vi "MTS_AutoZPos.vi"(0 "PH Dev":i32, 1 "OFlow Interv [s]":dbl, 2 "Accum Time [s]":dbl=0.1, 5 "PI System no.":i32, 11 "error in":errorcluster, 12 "Start Point":T1, 13 "Steps":i32=9, 14 "Step Width [um]":dbl=0.5) -> (4 "New Z":dbl, 6 "Counts":u32[](array[numeric]), 15 "error out":errorcluster)   [LabVIEW 2010]
panel:
  out "FiFo Overrun":bool
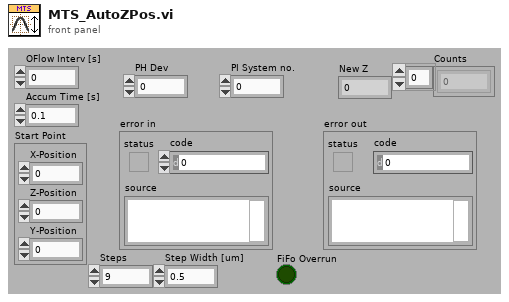
[diagram p1: front panel]
types:
  T1 = cluster{"X-Position":dbl, "Y-Position":dbl, "Z-Position":dbl}
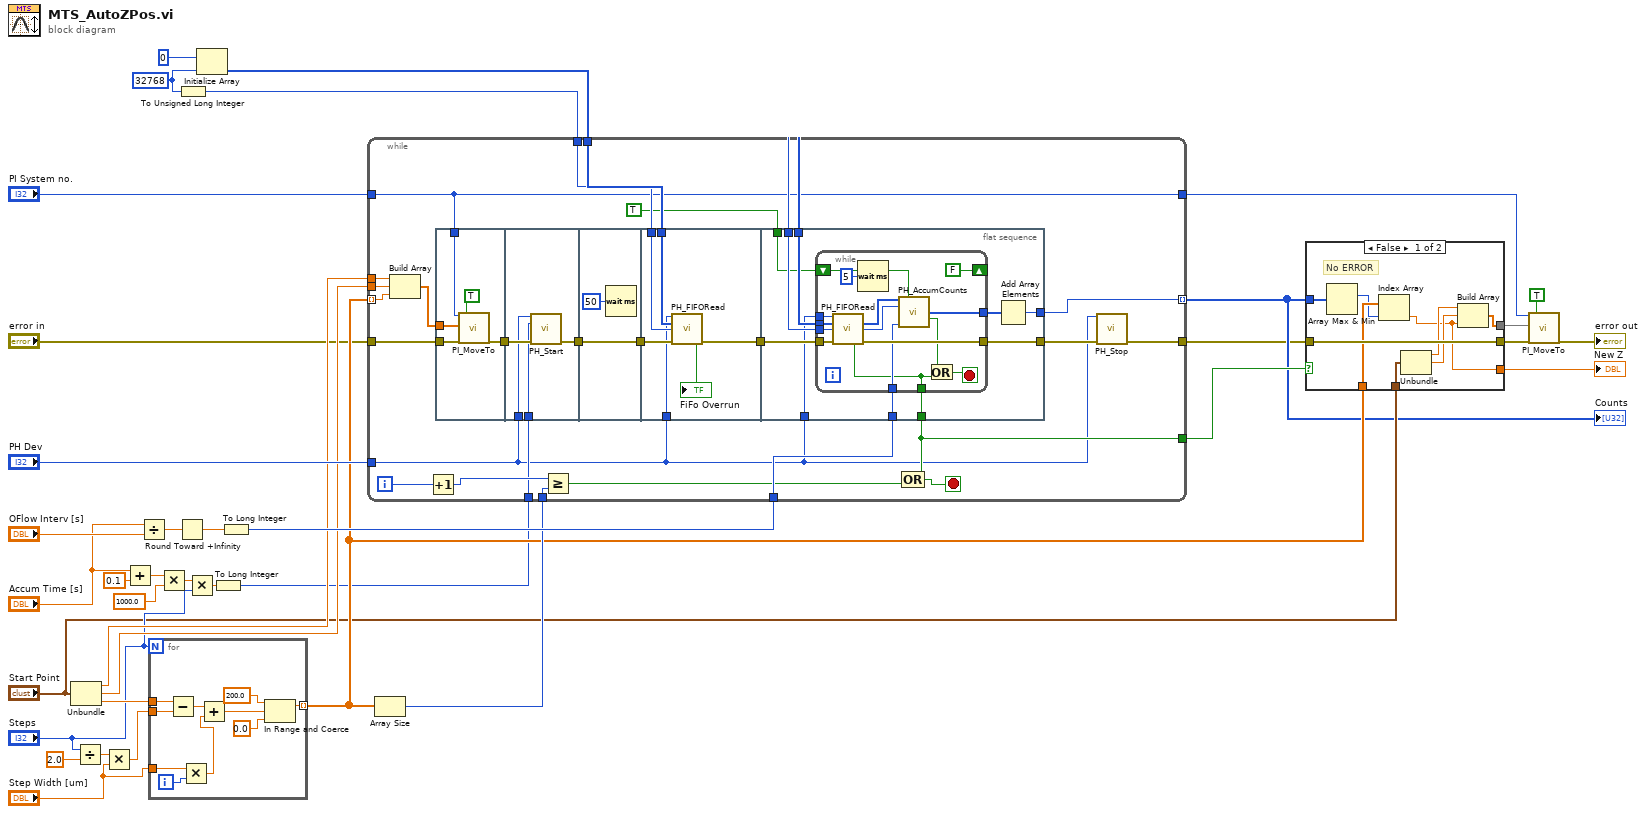
[diagram p0: block diagram]
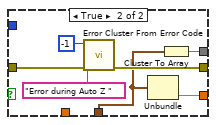
[diagram p2: hidden frame]
diagram:
  w38 = 32768 ("dimension size")
  n1 = Unbundle("Start Point") -> ("X-Position"=w21:dbl, "Y-Position"=w22:dbl, "Z-Position"=w25:dbl)
  n2 = Divide(x="Steps", y=2.0) -> (x/y=w28:dbl)
  n3 = Multiply(x=w28, y="Step Width [um]") -> (x*y=w24:dbl)
  n4 = Add(x="Accum Time [s]", y=0.1) -> (x+y=w17:dbl)
  n5 = Divide(x="Accum Time [s]", y="OFlow Interv [s]") -> (x/y=w31:dbl)
  n6 = for {
    N: "Steps" -> [_]
    tunnel: "Step Width [um]" -> [w47]
    tunnel: w25 -> [w46]
    tunnel: w24 -> [w43]
    tunnel: [w39] -> w8 mode=indexing
    i -> [w48]
    n7 = Subtract(x=w46, y=w43) -> (x-y=w42:dbl)
    n8 = Multiply(x=w47, y=w48) -> (x*y=w41:dbl)
    n9 = Add(x=w42, y=w41) -> (x+y=w40:dbl)
    n10 = In Range and Coerce(upper limit=200.0, x=w40, lower limit=0.0) -> (coerced(x)=w39:dbl)  [unwired: 1 out]
  }
  n11 = Multiply(x=w17, y=1000.0) -> (x*y=w15:dbl)
  n12 = Round Toward +Infinity(x=w31) -> (ceil(x): smallest int >= x=w30:dbl)
  n13 = To Unsigned Long Integer(number=w38) -> (unsigned 32bit integer=w35:u32)
  n14 = Multiply(x=w15, y="Steps") -> (x*y=w13:dbl)
  n15 = Initialize Array(u32 0, w38) -> (w36:u32[])
  n16 = To Long Integer(number=w13) -> (32bit integer=w2:i32)
  n17 = To Long Integer(number=w30) -> (32bit integer=w29:i32)
  n18 = Array Size(array=w8) -> (size(s)=w23:i32)
  n19 = while {
    tunnel: "error in" -> [w71]
    tunnel: w36 -> [w70]
    tunnel: w35 -> [w69]
    tunnel: "PH Dev" -> [w49]
    tunnel: [w50] -> w1
    tunnel: "PI System no." -> [w56]
    tunnel: w29 -> [w67]
    tunnel: w23 -> [w64]
    tunnel: w8 -> [w59] mode=indexing
    tunnel: w22 -> [w60]
    tunnel: w21 -> [w61]
    tunnel: [w57] -> w20
    tunnel: [w56] -> w10
    tunnel: [w55] -> w4 mode=indexing
    tunnel: w2 -> [w52]
    i -> [w66]
    stop <- w63 stop-if-true
    n20 = Build Array(w61, w60, w59) -> (w58:dbl[])
    n21 = Increment(x=w66) -> (x+1=w65:i32)
    n22 = flat-sequence {
      tunnel: w71 -> [w78]
      tunnel: [w77] -> w54
      tunnel: w56 -> [w76]
      tunnel: w58 -> [w75]
      tunnel: w54 -> [w82]
      tunnel: [w81] -> w53
      tunnel: w52 -> [w80]
      tunnel: w49 -> [w79]
      tunnel: [w83] -> w73
      tunnel: w53 -> [w83]
      tunnel: w73 -> [w90]
      tunnel: w70 -> [w89]
      tunnel: w69 -> [w88]
      tunnel: w49 -> [w87]
      tunnel: [w86] -> w72
      tunnel: w70 -> [w99]
      tunnel: w69 -> [w98]
      tunnel: w49 -> [w97]
      tunnel: [w96] -> w51
      tunnel: w72 -> [w100]
      tunnel: TRUE ("Reset") -> [w95]
      tunnel: w67 -> [w93]
      tunnel: [w92] -> w55
      tunnel: [w91] -> w57
      frame #0 {
        n23 = call "PI_MoveTo.vi"("System no."=w76, "Target position"=w75, "error in"=w78, "Move"=TRUE) -> ("error out"=w77:errorcluster)  [unwired: 13 in, 2 out]
      }
      frame #1 {
        n24 = call "PH_Start.vi"("Device Index"=w79, "Acq. Time"=w80, "error in (no error)"=w82) -> ("error out"=w81:errorcluster)  [unwired: 11 in, 1 out]
      }
      frame #2 {
        n25 = Wait (ms)(milliseconds to wait=u32 50) -> ()  [unwired: 1 out]
      }
      frame #3 {
        n26 = call "PH_FIFORead.vi"("Device Index"=w87, "Buffer In"=w89, "Count"=w88, "error in (no error)"=w90) -> ("FiFo Overrun"=→"FiFo Overrun":bool, "error out"=w86:errorcluster)  [unwired: 7 in, 3 out]
      }
      frame #4 {
        n27 = while {
          tunnel: w100 -> [w115]
          tunnel: w99 -> [w114]
          tunnel: w98 -> [w113]
          tunnel: w97 -> [w112]
          tunnel: [w111] -> w96
          shift-right: [FALSE ("Reset")] -> _
          shift-left: w95 -> [w107]
          tunnel: [w105] -> w94
          tunnel: w93 -> [w104]
          tunnel: [w101] -> w91
          stop <- w102 stop-if-true
          n28 = call "PH_FIFORead.vi"("Device Index"=w112, "Buffer In"=w114, "Count"=w113, "error in (no error)"=w115) -> ("Buffer Out"=w109:u32[], "Data Count"=w110:i32, "FiFo Overrun"=w101:bool, "error out"=w111:errorcluster)  [unwired: 7 in, 1 out]
          n29 = Wait (ms)(milliseconds to wait=u32 5) -> ()  [unwired: 1 out]
          n30 = call "PH_AccumCounts.vi"("Data In"=w109, "Reset"=w107, "Data Count"=w110, "Acc X Overflows"=w104) -> ("Accum Counts"=w105:u32[], "Acc Time Ok"=w103:bool)  [unwired: 7 in, 3 out]
          n31 = Or(x=w103, y=w101) -> (x .or. y?=w102:bool)
        }
        n32 = Add Array Elements(numeric array=w94) -> (sum=w92:u32)
      }
    }
    n33 = Greater Or Equal?(x=w65, y=w64) -> (x >= y?=w62:bool)
    n34 = Compound Arithmetic op=OR(w57, w62) -> (w63:bool)
    n35 = call "PH_Stop.vi"("Device Index"=w49, "error in (no error)"=w51) -> ("error out"=w50:errorcluster)  [unwired: 12 in, 1 out]
  }
  "Counts" <- w4
  n36 = case shown="False" w20 {
    tunnel: w1 -> [w124 w131]
    tunnel: [w124 w130] -> w12
    tunnel: w4 -> [w123 _]
    tunnel: w8 -> [w122 _]
    tunnel: "Start Point" -> [w120 w126]
    tunnel: [w117 w127] -> w6
    tunnel: [w116 w125] -> w5
    frame False {
      # "No ERROR"
      n37 = Array Max & Min(array=w123) -> (max index (indices)=w121:i32)  [unwired: 3 out]
      n38 = Index Array(array=w122, index=w121) -> (element=w116:dbl)
      n39 = Unbundle(w120) -> ("X-Position"=w119:dbl, "Y-Position"=w118:dbl)  [unwired: 1 out]
      n40 = Build Array(w119, w118, w116) -> (w117:dbl[])
    }
    frame True {
      n41 = call <vilib>:"Error Cluster From Error Code.vi"("error in (no error)"=w131, "error message (\"\")"="Error during Auto Z " ("error message (\"\")"), "error code (0)"=-1) -> ("error out"=w130:errorcluster)  [unwired: 6 in]
      n42 = Unbundle(w126) -> ("Z-Position"=w125:dbl)  [unwired: 2 out]
      n43 = Cluster To Array(cluster=w126) -> (array=w127:dbl[])
    }
  }
  "New Z" <- w5
  n44 = call "PI_MoveTo.vi"("System no."=w10, "Target position"=w6, "error in"=w12, "Move"=TRUE) -> ("error out"=→"error out":errorcluster)  [unwired: 13 in, 2 out]
